vi "p_observer.vi"(0 "y":dbl, 3 "Kp":dbl, 4 "dt":dbl=1.0, 5 "Reset":bool) -> (7 "y_dot":dbl)   [LabVIEW 2021]
uses:
  <vilib>/ptbypt/NI_PtbyPt.lvlib
panel:
  # "desired signal"
  # "substratction"
  # "Integrator"
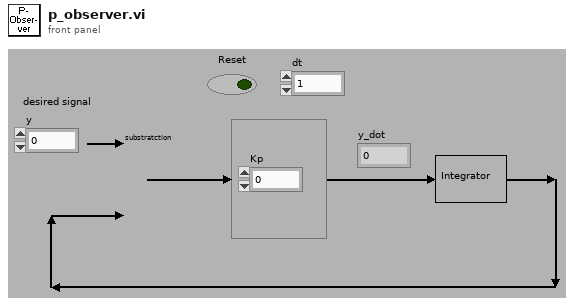
[diagram p1: front panel]
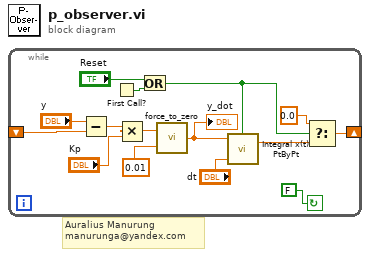
[diagram p0: block diagram]
diagram:
  # "Auralius Manurung\nmanurunga@yandex.com"
  n1 = while {
    shift-right: [w4] -> _
    shift-left: _ -> [w14]
    stop <- FALSE continue-if-true
    n2 = Subtract(x="y", y=w14) -> (x-y=w9:dbl)
    n3 = First Call?() -> (First Call?: T/F=w11:bool)
    n4 = Multiply(x=w9, y="Kp") -> (x*y=w3:dbl)
    n5 = Or(x="Reset", y=w11) -> (x .or. y?=w5:bool)
    n6 = call "force_to_zero.vi"("Epsilon"=0.01, "Input"=w3) -> ("Output"=w2:dbl)
    "y_dot" <- w2
    n7 = call <vilib>:"Integral x(t) PtByPt.vi"("initialize"=w5, "dt"="dt", "x"=w2) -> ("integral x(t)"=w6:dbl)  [unwired: 1 in, 1 out]
    n8 = Select(t=0.0, s=w5, f=w6) -> (s? t:f=w4:dbl)
  }
